vi "user interface.vi"() -> ()   [LabVIEW 2014]
panel:
  out "stage":dbl
  in  "start":cluster{"String":string, "play":bool}={"String"="\nTomb Of The Mask", "play"=FALSE}
  in  "quit":bool
  in  "next stage or choosing stage":T1
  in  "choosing stage":T2
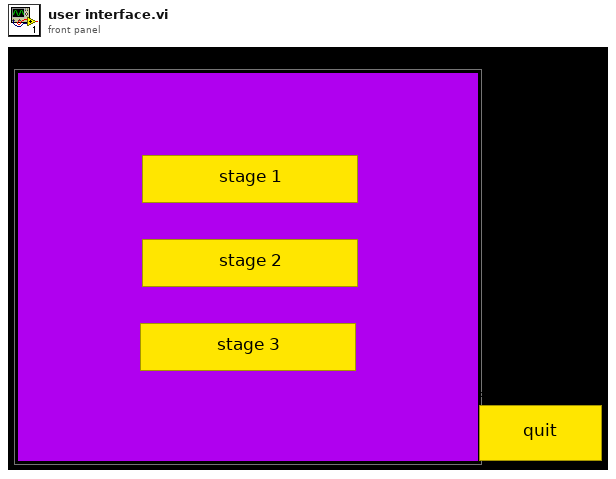
[diagram p1: front panel]
types:
  T1 = cluster{"next stage ":bool, "back":bool, "Boolean":bool, "Boolean 2":bool, "Boolean 3":bool}
  T2 = cluster{"stage 1":bool, "stage 2":bool, "stsage 3":bool}
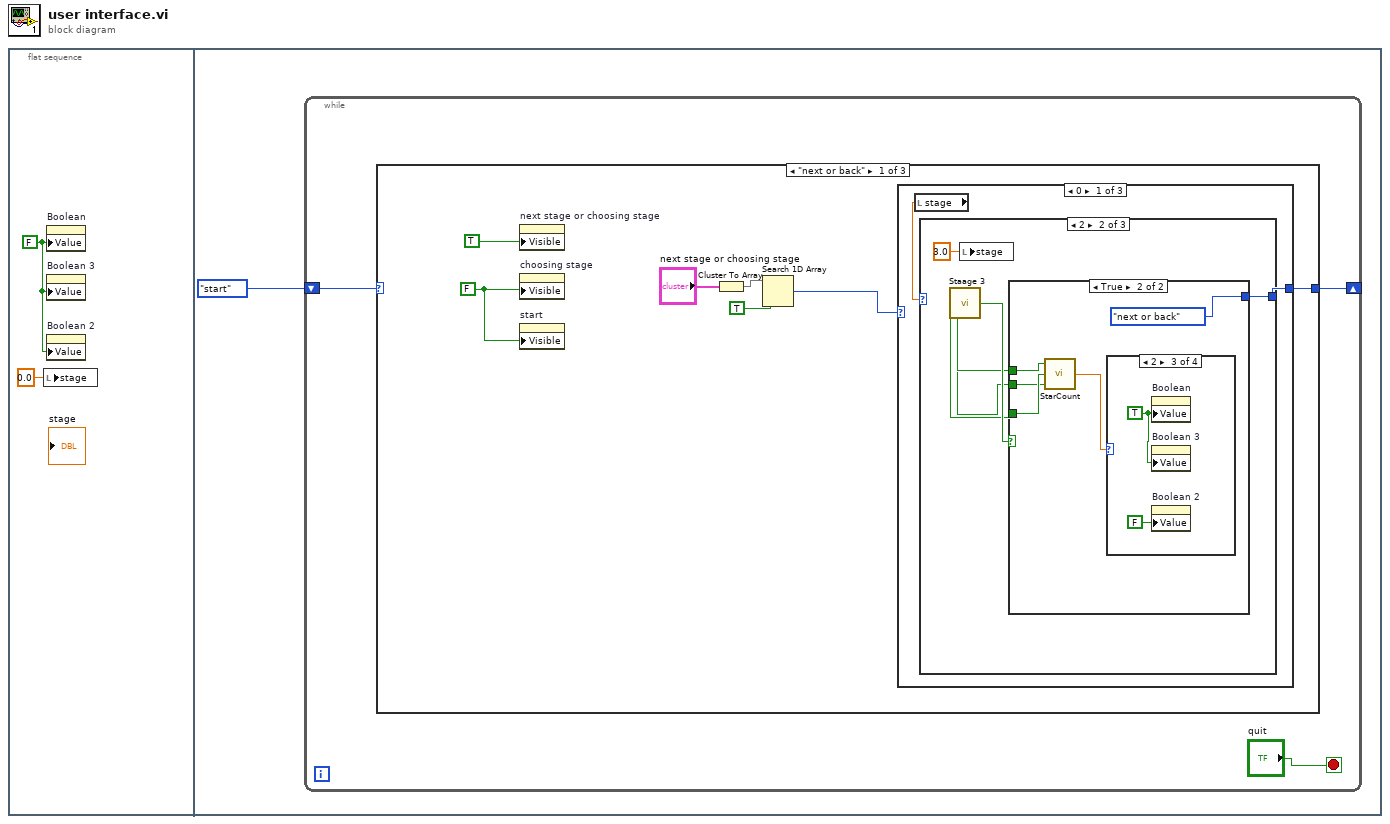
[diagram p0: block diagram]
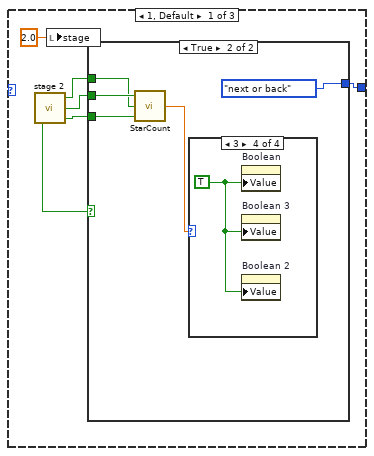
[diagram p2: hidden frame]
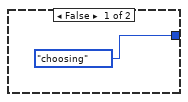
[diagram p3: hidden frame]
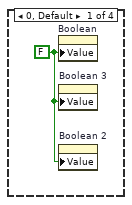
[diagram p4: hidden frame]
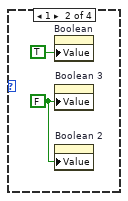
[diagram p5: hidden frame]
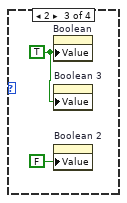
[diagram p6: hidden frame]
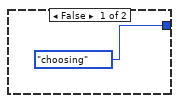
[diagram p7: hidden frame]
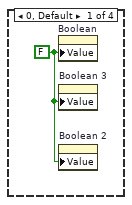
[diagram p8: hidden frame]
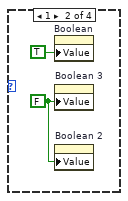
[diagram p9: hidden frame]
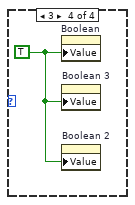
[diagram p10: hidden frame]
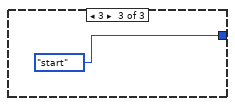
[diagram p11: hidden frame]
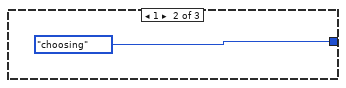
[diagram p12: hidden frame]
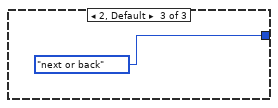
[diagram p13: hidden frame]
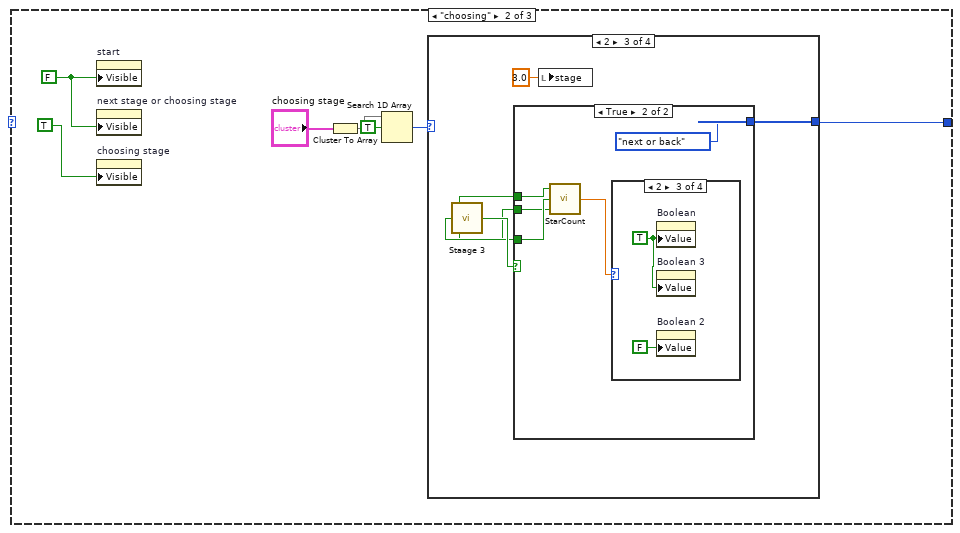
[diagram p14: hidden frame]
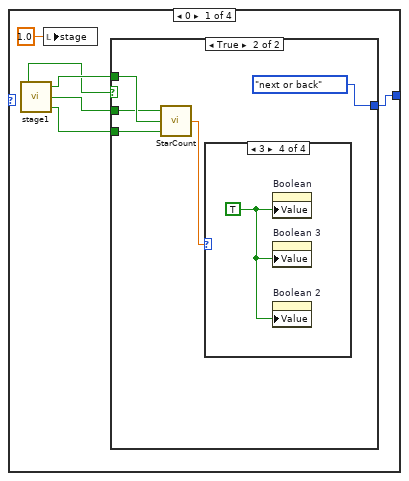
[diagram p15: hidden frame]
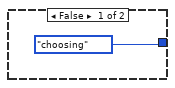
[diagram p16: hidden frame]
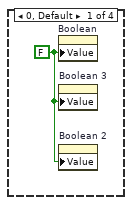
[diagram p17: hidden frame]
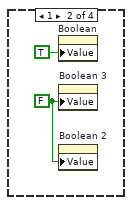
[diagram p18: hidden frame]
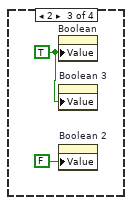
[diagram p19: hidden frame]
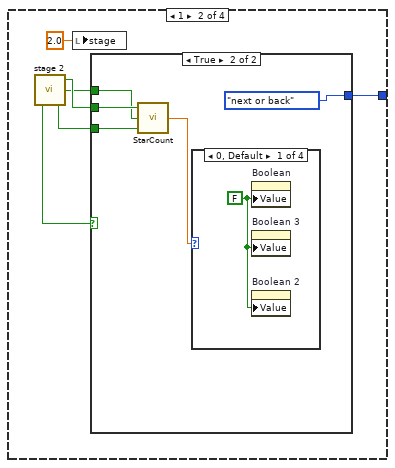
[diagram p20: hidden frame]
diagram:
  n1 = flat-sequence {
    frame #0 {
      w1 = FALSE ("Value")
      n2 = local write "stage"(0.0 ("stage")) -> ()
      n3 = property on="Boolean" class="Bool (strict)"("Value"=w1) -> ()  [unwired: 2 in, 2 out]
      n4 = property on="Boolean 3" class="Bool (strict)"("Value"=w1) -> ()  [unwired: 2 in, 2 out]
      n5 = property on="Boolean 2" class="Bool (strict)"("Value"=w1) -> ()  [unwired: 2 in, 2 out]
    }
    frame #1 {
      n6 = while {
        shift-right: [w5] -> _
        shift-left: enum16{"next or back", "choosing", "start"}."start" ("Enum") -> [w6]
        stop <- "quit" stop-if-true
        n7 = case shown="\"next or back\"" w6 {
          tunnel: [w7 w55 w117] -> w5
          frame "next or back" {
            w12 = FALSE ("Visible")
            n8 = property on="next stage or choosing stage" class="Clust"("Visible"=TRUE) -> ()  [unwired: 2 in, 2 out]
            n9 = property on="choosing stage" class="Clust"("Visible"=w12) -> ()  [unwired: 2 in, 2 out]
            n10 = property on="start" class="Clust"("Visible"=w12) -> ()  [unwired: 2 in, 2 out]
            n11 = Cluster To Array(cluster="next stage or choosing stage") -> (array=w10:bool[])
            n12 = Search 1D Array(1D array=w10, element=TRUE) -> (index of element=w8:i32)  [unwired: 1 in]
            n13 = case shown="0" w8 {
              tunnel: [w14 enum16{"next or back", "choosing", "start"}."choosing" ("Enum") enum16{"next or back", "choosing", "start"}."next or back" ("Enum")] -> w7
              frame 0 {
                n14 = local read "stage"() -> (w15:dbl)
                n15 = case shown="2" w15 {
                  tunnel: [w17 w39 enum16{"next or back", "choosing", "start"}."start" ("Enum")] -> w14
                  frame 1, Default {
                    n16 = call "stage 2.vi"() -> ("pass"=w21:bool, "Boolean 5"=w20:bool, "Boolean 7"=w19:bool, "Boolean 8"=w18:bool)
                    n17 = local write "stage"(2.0 ("stage")) -> ()
                    n18 = case shown="True" w21 {
                      tunnel: w19 -> [_ w27]
                      tunnel: w20 -> [_ w26]
                      tunnel: w18 -> [_ w25]
                      tunnel: [enum16{"next or back", "choosing", "start"}."choosing" ("Enum") enum16{"next or back", "choosing", "start"}."next or back" ("Enum")] -> w17
                      frame False {
                      }
                      frame True {
                        n19 = call "StarCount.vi"("Boolean 2"=w25, "Boolean"=w26, "Boolean 3"=w27) -> ("Numeric"=w24:dbl)
                        n20 = case shown="3" w24 {
                          frame 0, Default {
                            w28 = FALSE ("Value")
                            n21 = property on="Boolean" class="Bool (strict)"("Value"=w28) -> ()  [unwired: 2 in, 2 out]
                            n22 = property on="Boolean 3" class="Bool (strict)"("Value"=w28) -> ()  [unwired: 2 in, 2 out]
                            n23 = property on="Boolean 2" class="Bool (strict)"("Value"=w28) -> ()  [unwired: 2 in, 2 out]
                          }
                          frame 1 {
                            w29 = FALSE ("Value")
                            n24 = property on="Boolean" class="Bool (strict)"("Value"=TRUE) -> ()  [unwired: 2 in, 2 out]
                            n25 = property on="Boolean 3" class="Bool (strict)"("Value"=w29) -> ()  [unwired: 2 in, 2 out]
                            n26 = property on="Boolean 2" class="Bool (strict)"("Value"=w29) -> ()  [unwired: 2 in, 2 out]
                          }
                          frame 2 {
                            w32 = TRUE ("Value")
                            n27 = property on="Boolean" class="Bool (strict)"("Value"=w32) -> ()  [unwired: 2 in, 2 out]
                            n28 = property on="Boolean 3" class="Bool (strict)"("Value"=w32) -> ()  [unwired: 2 in, 2 out]
                            n29 = property on="Boolean 2" class="Bool (strict)"("Value"=FALSE) -> ()  [unwired: 2 in, 2 out]
                          }
                          frame 3 {
                            w33 = TRUE ("Value")
                            n30 = property on="Boolean" class="Bool (strict)"("Value"=w33) -> ()  [unwired: 2 in, 2 out]
                            n31 = property on="Boolean 3" class="Bool (strict)"("Value"=w33) -> ()  [unwired: 2 in, 2 out]
                            n32 = property on="Boolean 2" class="Bool (strict)"("Value"=w33) -> ()  [unwired: 2 in, 2 out]
                          }
                        }
                      }
                    }
                  }
                  frame 2 {
                    n33 = call "Staage 3.vi"() -> ("pass"=w38:bool, "Boolean 5"=w35:bool, "Boolean 7"=w36:bool, "Boolean 8"=w37:bool)
                    n34 = local write "stage"(3.0 ("stage")) -> ()
                    n35 = case shown="True" w38 {
                      tunnel: [enum16{"next or back", "choosing", "start"}."choosing" ("Enum") enum16{"next or back", "choosing", "start"}."next or back" ("Enum")] -> w39
                      tunnel: w37 -> [_ w43]
                      tunnel: w36 -> [_ w42]
                      tunnel: w35 -> [_ w41]
                      frame False {
                      }
                      frame True {
                        n36 = call "StarCount.vi"("Boolean 2"=w41, "Boolean"=w42, "Boolean 3"=w43) -> ("Numeric"=w45:dbl)
                        n37 = case shown="2" w45 {
                          frame 0, Default {
                            w46 = FALSE ("Value")
                            n38 = property on="Boolean" class="Bool (strict)"("Value"=w46) -> ()  [unwired: 2 in, 2 out]
                            n39 = property on="Boolean 3" class="Bool (strict)"("Value"=w46) -> ()  [unwired: 2 in, 2 out]
                            n40 = property on="Boolean 2" class="Bool (strict)"("Value"=w46) -> ()  [unwired: 2 in, 2 out]
                          }
                          frame 1 {
                            w47 = FALSE ("Value")
                            n41 = property on="Boolean" class="Bool (strict)"("Value"=TRUE) -> ()  [unwired: 2 in, 2 out]
                            n42 = property on="Boolean 3" class="Bool (strict)"("Value"=w47) -> ()  [unwired: 2 in, 2 out]
                            n43 = property on="Boolean 2" class="Bool (strict)"("Value"=w47) -> ()  [unwired: 2 in, 2 out]
                          }
                          frame 2 {
                            w50 = TRUE ("Value")
                            n44 = property on="Boolean" class="Bool (strict)"("Value"=w50) -> ()  [unwired: 2 in, 2 out]
                            n45 = property on="Boolean 3" class="Bool (strict)"("Value"=w50) -> ()  [unwired: 2 in, 2 out]
                            n46 = property on="Boolean 2" class="Bool (strict)"("Value"=FALSE) -> ()  [unwired: 2 in, 2 out]
                          }
                          frame 3 {
                            w51 = TRUE ("Value")
                            n47 = property on="Boolean" class="Bool (strict)"("Value"=w51) -> ()  [unwired: 2 in, 2 out]
                            n48 = property on="Boolean 3" class="Bool (strict)"("Value"=w51) -> ()  [unwired: 2 in, 2 out]
                            n49 = property on="Boolean 2" class="Bool (strict)"("Value"=w51) -> ()  [unwired: 2 in, 2 out]
                          }
                        }
                      }
                    }
                  }
                  frame 3 {
                  }
                }
              }
              frame 1 {
              }
              frame 2, Default {
              }
            }
          }
          frame "choosing" {
            w60 = FALSE ("Visible")
            n50 = property on="start" class="Clust"("Visible"=w60) -> ()  [unwired: 2 in, 2 out]
            n51 = property on="next stage or choosing stage" class="Clust"("Visible"=w60) -> ()  [unwired: 2 in, 2 out]
            n52 = property on="choosing stage" class="Clust"("Visible"=TRUE) -> ()  [unwired: 2 in, 2 out]
            n53 = Cluster To Array(cluster="choosing stage") -> (array=w58:bool[])
            n54 = Search 1D Array(1D array=w58, element=TRUE) -> (index of element=w56:i32)  [unwired: 1 in]
            n55 = case shown="2" w56 {
              tunnel: [w64 w80 w98 enum16{"next or back", "choosing", "start"}."choosing" ("Enum")] -> w55
              frame 0 {
                n56 = call "stage1.vi"() -> ("pass"=w63:bool, "Boolean 5"=w65:bool, "Boolean 8"=w62:bool, "Boolean 7"=w66:bool)
                n57 = local write "stage"(1.0 ("stage")) -> ()
                n58 = case shown="True" w63 {
                  tunnel: w66 -> [_ w73]
                  tunnel: w65 -> [_ w72]
                  tunnel: w62 -> [_ w71]
                  tunnel: [enum16{"next or back", "choosing", "start"}."choosing" ("Enum") enum16{"next or back", "choosing", "start"}."next or back" ("Enum")] -> w64
                  frame False {
                  }
                  frame True {
                    n59 = call "StarCount.vi"("Boolean 2"=w73, "Boolean"=w72, "Boolean 3"=w71) -> ("Numeric"=w69:dbl)
                    n60 = case shown="3" w69 {
                      frame 0, Default {
                        w74 = FALSE ("Value")
                        n61 = property on="Boolean" class="Bool (strict)"("Value"=w74) -> ()  [unwired: 2 in, 2 out]
                        n62 = property on="Boolean 3" class="Bool (strict)"("Value"=w74) -> ()  [unwired: 2 in, 2 out]
                        n63 = property on="Boolean 2" class="Bool (strict)"("Value"=w74) -> ()  [unwired: 2 in, 2 out]
                      }
                      frame 1 {
                        w75 = FALSE ("Value")
                        n64 = property on="Boolean" class="Bool (strict)"("Value"=TRUE) -> ()  [unwired: 2 in, 2 out]
                        n65 = property on="Boolean 3" class="Bool (strict)"("Value"=w75) -> ()  [unwired: 2 in, 2 out]
                        n66 = property on="Boolean 2" class="Bool (strict)"("Value"=w75) -> ()  [unwired: 2 in, 2 out]
                      }
                      frame 2 {
                        w78 = TRUE ("Value")
                        n67 = property on="Boolean" class="Bool (strict)"("Value"=w78) -> ()  [unwired: 2 in, 2 out]
                        n68 = property on="Boolean 3" class="Bool (strict)"("Value"=w78) -> ()  [unwired: 2 in, 2 out]
                        n69 = property on="Boolean 2" class="Bool (strict)"("Value"=FALSE) -> ()  [unwired: 2 in, 2 out]
                      }
                      frame 3 {
                        w79 = TRUE ("Value")
                        n70 = property on="Boolean" class="Bool (strict)"("Value"=w79) -> ()  [unwired: 2 in, 2 out]
                        n71 = property on="Boolean 3" class="Bool (strict)"("Value"=w79) -> ()  [unwired: 2 in, 2 out]
                        n72 = property on="Boolean 2" class="Bool (strict)"("Value"=w79) -> ()  [unwired: 2 in, 2 out]
                      }
                    }
                  }
                }
              }
              frame 1 {
                n73 = call "stage 2.vi"() -> ("pass"=w84:bool, "Boolean 5"=w83:bool, "Boolean 7"=w82:bool, "Boolean 8"=w81:bool)
                n74 = local write "stage"(2.0 ("stage")) -> ()
                n75 = case shown="True" w84 {
                  tunnel: w83 -> [_ w91]
                  tunnel: w82 -> [_ w90]
                  tunnel: w81 -> [_ w89]
                  tunnel: [enum16{"next or back", "choosing", "start"}."choosing" ("Enum") enum16{"next or back", "choosing", "start"}."next or back" ("Enum")] -> w80
                  frame False {
                  }
                  frame True {
                    n76 = call "StarCount.vi"("Boolean 2"=w89, "Boolean"=w90, "Boolean 3"=w91) -> ("Numeric"=w88:dbl)
                    n77 = case shown="0, Default" w88 {
                      frame 0, Default {
                        w92 = FALSE ("Value")
                        n78 = property on="Boolean" class="Bool (strict)"("Value"=w92) -> ()  [unwired: 2 in, 2 out]
                        n79 = property on="Boolean 3" class="Bool (strict)"("Value"=w92) -> ()  [unwired: 2 in, 2 out]
                        n80 = property on="Boolean 2" class="Bool (strict)"("Value"=w92) -> ()  [unwired: 2 in, 2 out]
                      }
                      frame 1 {
                        w93 = FALSE ("Value")
                        n81 = property on="Boolean" class="Bool (strict)"("Value"=TRUE) -> ()  [unwired: 2 in, 2 out]
                        n82 = property on="Boolean 3" class="Bool (strict)"("Value"=w93) -> ()  [unwired: 2 in, 2 out]
                        n83 = property on="Boolean 2" class="Bool (strict)"("Value"=w93) -> ()  [unwired: 2 in, 2 out]
                      }
                      frame 2 {
                        w96 = TRUE ("Value")
                        n84 = property on="Boolean" class="Bool (strict)"("Value"=w96) -> ()  [unwired: 2 in, 2 out]
                        n85 = property on="Boolean 3" class="Bool (strict)"("Value"=w96) -> ()  [unwired: 2 in, 2 out]
                        n86 = property on="Boolean 2" class="Bool (strict)"("Value"=FALSE) -> ()  [unwired: 2 in, 2 out]
                      }
                      frame 3 {
                        w97 = TRUE ("Value")
                        n87 = property on="Boolean" class="Bool (strict)"("Value"=w97) -> ()  [unwired: 2 in, 2 out]
                        n88 = property on="Boolean 3" class="Bool (strict)"("Value"=w97) -> ()  [unwired: 2 in, 2 out]
                        n89 = property on="Boolean 2" class="Bool (strict)"("Value"=w97) -> ()  [unwired: 2 in, 2 out]
                      }
                    }
                  }
                }
              }
              frame 2 {
                n90 = call "Staage 3.vi"() -> ("pass"=w102:bool, "Boolean 5"=w99:bool, "Boolean 7"=w100:bool, "Boolean 8"=w101:bool)
                n91 = case shown="True" w102 {
                  tunnel: w101 -> [_ w109]
                  tunnel: w100 -> [_ w108]
                  tunnel: w99 -> [_ w107]
                  tunnel: [enum16{"next or back", "choosing", "start"}."choosing" ("Enum") enum16{"next or back", "choosing", "start"}."next or back" ("Enum")] -> w98
                  frame False {
                  }
                  frame True {
                    n92 = call "StarCount.vi"("Boolean 2"=w107, "Boolean"=w108, "Boolean 3"=w109) -> ("Numeric"=w106:dbl)
                    n93 = case shown="2" w106 {
                      frame 0, Default {
                        w110 = FALSE ("Value")
                        n94 = property on="Boolean" class="Bool (strict)"("Value"=w110) -> ()  [unwired: 2 in, 2 out]
                        n95 = property on="Boolean 3" class="Bool (strict)"("Value"=w110) -> ()  [unwired: 2 in, 2 out]
                        n96 = property on="Boolean 2" class="Bool (strict)"("Value"=w110) -> ()  [unwired: 2 in, 2 out]
                      }
                      frame 1 {
                        w111 = FALSE ("Value")
                        n97 = property on="Boolean" class="Bool (strict)"("Value"=TRUE) -> ()  [unwired: 2 in, 2 out]
                        n98 = property on="Boolean 3" class="Bool (strict)"("Value"=w111) -> ()  [unwired: 2 in, 2 out]
                        n99 = property on="Boolean 2" class="Bool (strict)"("Value"=w111) -> ()  [unwired: 2 in, 2 out]
                      }
                      frame 2 {
                        w114 = TRUE ("Value")
                        n100 = property on="Boolean" class="Bool (strict)"("Value"=w114) -> ()  [unwired: 2 in, 2 out]
                        n101 = property on="Boolean 3" class="Bool (strict)"("Value"=w114) -> ()  [unwired: 2 in, 2 out]
                        n102 = property on="Boolean 2" class="Bool (strict)"("Value"=FALSE) -> ()  [unwired: 2 in, 2 out]
                      }
                      frame 3 {
                        w115 = TRUE ("Value")
                        n103 = property on="Boolean" class="Bool (strict)"("Value"=w115) -> ()  [unwired: 2 in, 2 out]
                        n104 = property on="Boolean 3" class="Bool (strict)"("Value"=w115) -> ()  [unwired: 2 in, 2 out]
                        n105 = property on="Boolean 2" class="Bool (strict)"("Value"=w115) -> ()  [unwired: 2 in, 2 out]
                      }
                    }
                  }
                }
                n106 = local write "stage"(3.0 ("stage")) -> ()
              }
              frame 3, Default {
              }
            }
          }
          frame "start", Default {
            w124 = FALSE ("Visible")
            n107 = property on="start" class="Clust"("Visible"=TRUE) -> ()  [unwired: 2 in, 2 out]
            n108 = property on="next stage or choosing stage" class="Clust"("Visible"=w124) -> ()  [unwired: 2 in, 2 out]
            n109 = property on="choosing stage" class="Clust"("Visible"=w124) -> ()  [unwired: 2 in, 2 out]
            n110 = Unbundle By Name("start") -> ("play"=w122:bool)
            n111 = Equal?(x=w122, y=TRUE) -> (x = y?=w120:bool)
            n112 = Select(t=enum16{"next or back", "choosing", "start"}."choosing" ("Enum"), s=w120, f=enum16{"next or back", "choosing", "start"}."start" ("Enum")) -> (s? t:f=w117:enum16{"next or back", "choosing", "start"})
          }
        }
      }
    }
  }
